vi "Best fit axis-aligned ellipse.vi"(0 "x array":dbl[](array[numeric]), 1 "y array":dbl[](array[numeric])) -> (2 "x centre":dbl, 3 "y centre":dbl, 4 "x radius":dbl, 5 "y radius":dbl)   [LabVIEW 2014]
doc: "Finds the best fit axis-aligned ellipse using a non-linear least squares method. Input arrays (corresponding values of x and y) must have a minimum of 4 values each"
uses:
  <vilib>/Analysis/baseanly.llb/Real A x B.vi
  <vilib>/Analysis/baseanly.llb/A x Vector.vi
  <vilib>/Analysis/Matrix/Numeric/Conversions/Array To Matrix - RA2.vi
  <vilib>/Analysis/baseanly.llb/Real Inverse Matrix.vi
  <vilib>/Analysis/Matrix/NI_Matrix.lvlib
  <vilib>/Analysis/NI_AALBase.lvlib
panel:
  # "Paul Nathan 24/06/2015"
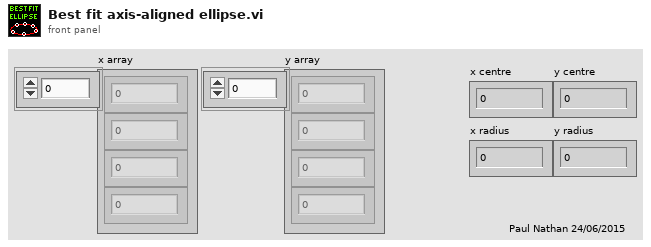
[diagram p1: front panel]
types:
  T1 = typedef "NI_Matrix.lvlib/RealMatrix.ctl" = dbl[][]
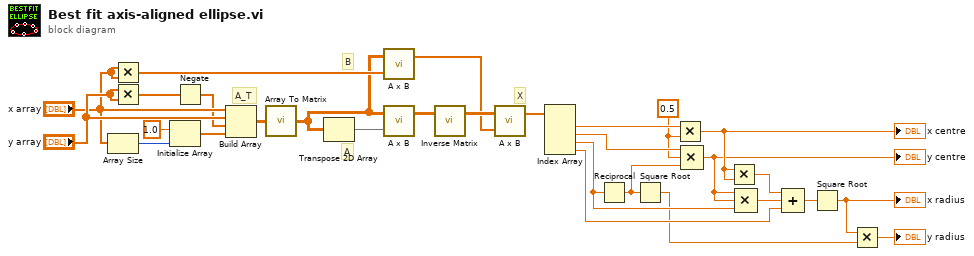
[diagram p0: block diagram]
diagram:
  w18 = 0.5 ("y")
  # "A_T"
  # "X"
  # "A"
  # "B"
  n1 = Array Size(array="x array") -> (size(s)=w29:i32)
  n2 = Multiply(x="x array", y="x array") -> (x*y=w12:dbl[])
  n3 = Multiply(x="y array", y="y array") -> (x*y=w11:dbl[])
  n4 = Initialize Array(1.0 ("element"), w29) -> (w13:dbl[])
  n5 = Negate(x=w11) -> (-x=w10:dbl[])
  n6 = Build Array("x array", "y array", w10, w13) -> (w25:dbl[][])
  n7 = call-poly <vilib>:"Array To Matrix.vi"("Real 2D Array"=w25) -> ("Real Matrix"=w1:T1)
  n8 = Transpose 2D Array(2D array=w1) -> (transposed array=w2:T1)
  n9 = call-poly <vilib>:"A x B.vi"("Vector"=w12, "A"=w1) -> ("A x Vector"=w22:dbl[])  [unwired: 1 out]
  n10 = call-poly <vilib>:"A x B.vi"("B"=w2, "A"=w1) -> ("A x B"=w24:T1)  [unwired: 1 out]
  n11 = call-poly <vilib>:"Inverse Matrix.vi"("Input Matrix"=w24) -> ("Inverse Matrix"=w23:T1)  [unwired: 1 in, 1 out]
  n12 = call-poly <vilib>:"A x B.vi"("Vector"=w22, "A"=w23) -> ("A x Vector"=w21:dbl[])  [unwired: 1 out]
  n13 = Index Array(array=w21) -> (element #1=w20:dbl, element #2=w19:dbl, element #3=w7:dbl, element #4=w9:dbl)  [unwired: 4 in]
  n14 = Reciprocal(x=w7) -> (1/x=w8:dbl)
  n15 = Square Root(x=w8) -> (sqrt(x)=w4:dbl)
  n16 = Multiply(x=w20, y=w18) -> (x*y=w17:dbl)
  "x centre" <- w17
  n17 = Compound Arithmetic op=MULTIPLY(w19, w18, w8) -> (w16:dbl)
  "y centre" <- w16
  n18 = Multiply(x=w17, y=w17) -> (x*y=w15:dbl)
  n19 = Compound Arithmetic op=MULTIPLY(w16, w16, w7) -> (w6:dbl)
  n20 = Compound Arithmetic op=ADD(w15, w6, w9) -> (w14:dbl)
  n21 = Square Root(x=w14) -> (sqrt(x)=w5:dbl)
  "x radius" <- w5
  n22 = Multiply(x=w5, y=w4) -> (x*y=→"y radius":dbl)
